vi "test uSec.vi"() -> ()   [LabVIEW 2019]
panel:
  out "Tick Count(uSec)":u32
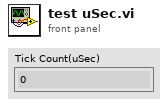
[diagram p1: front panel]
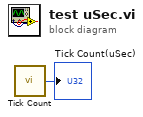
[diagram p0: block diagram]
diagram:
  n1 = call "Tick Count"() -> ("Tick Count(uSec)"=→"Tick Count(uSec)":u32)
